vi "_Q. LocatorCallback.vi"(4 "context in":variant, 5 "objref":refnum<vi>) -> (1 "context out":variant, 2 "traverse flags":i32)   [LabVIEW 2020]
uses:
  <vilib>/Utility/miscctls.llb/LVPoint32TypeDef.ctl
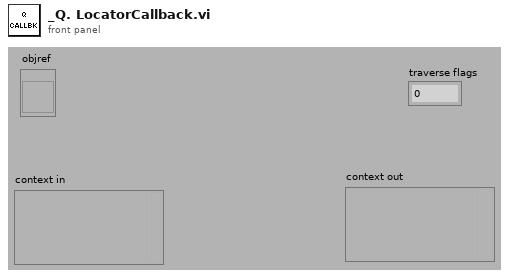
[diagram p1: front panel]
types:
  T1 = typedef "LVPoint32TypeDef.ctl" = cluster{"Horizontal":i32, "Vertical":i32}
  T2 = typedef "LVRectTypeDef.ctl" = cluster{"Left":i16, "Top":i16, "Right":i16, "Bottom":i16}
  T3 = cluster{"Coords":T1, "objref":refnum<vi>, "pt in rect":bool}
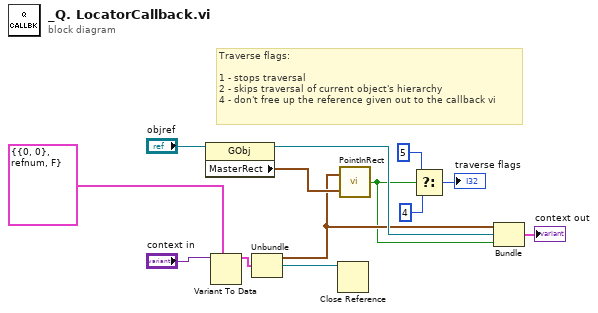
[diagram p0: block diagram]
diagram:
  # "Traverse flags:\n\n1\t- stops traversal \n2\t- skips traversal of current object's hierarchy\n4 - don't free up the reference given out to the callback vi"
  n1 = property class="GObj"(reference="objref") -> (reference out=w8:refnum<vi>, "MasterRect"=w9:T2)  [unwired: 1 in, 1 out]
  n2 = Variant To Data(type=cluster{"Coords":T1, refnum<vi>, "Found?":bool} {"Coords"={"Horizontal"=0, "Vertical"=0}, refnum, "Found?"=FALSE}, Variant="context in") -> (data=w11:cluster{"Coords":T1, refnum<vi>, "Found?":bool})  [unwired: 1 in, 1 out]
  n3 = Unbundle(w11) -> ("Coords"=w7:T1, w1:refnum<vi>)  [unwired: 1 out]
  n4 = Close Reference(reference=w1) -> ()  [unwired: 1 in, 1 out]
  n5 = call <vilib>:"PointInRect.vi"("rect"=w9, "point"=w7) -> ("pt in rect"=w2:bool)
  n6 = Select(t=5 ("Traverse Flags"), s=w2, f=4 ("Traverse Flags")) -> (s? t:f=→"traverse flags":i32)
  n7 = Bundle("Coords"=w7, "objref"=w8, "pt in rect"=w2) -> (→"context out":T3)  [unwired: 1 in]
